vi "Initialize New.vi"(4 "Error In":errorcluster, 7 "Config Data_DB in":refnum<class "Config Data_DB.lvclass">) -> (0 "Error Out":errorcluster, 3 "Config Data_DB out":refnum<class "Config Data_DB.lvclass">)   [LabVIEW 2014, in "Config Data.lvlib" / "Config Data_DB.lvclass"]
uses:
  Config Data_DB.lvclass
  Config Data_DB.lvclass/Config Data_DB.ctl
  Config Data.lvclass
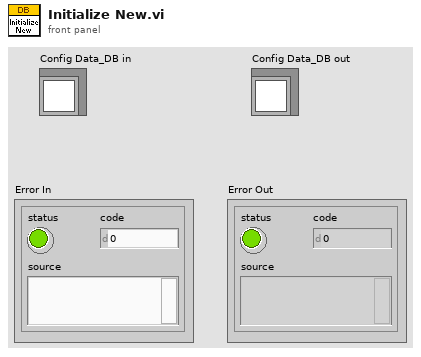
[diagram p1: front panel]
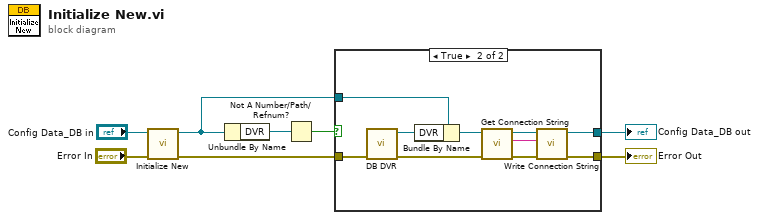
[diagram p0: block diagram]
diagram:
  n1 = call-parent "Initialize New.vi"("Error In"="Error In", "Config Data in"="Config Data_DB in") -> ("Error Out"=w3:errorcluster, "Config Data out"=w4:refnum<class "Config Data_DB.lvclass">)  [unwired: 4 in]
  n2 = Unbundle By Name(w4) -> ("DVR"=w6:refnum<data-value>)
  n3 = Not A Number/Path/Refnum?(number/path/refnum=w6) -> (NaN/Path/Refnum?=w5:bool)
  n4 = case shown="True" w5 {
    tunnel: w4 -> [w10 w20]
    tunnel: [w10 w12] -> w2
    tunnel: w3 -> [w9 w19]
    tunnel: [w9 w11] -> w1
    frame False {
    }
    frame True {
      n5 = call "DB DVR.vi"("Error In"=w19) -> ("Error Out"=w16:errorcluster, "DVR"=w18:refnum<data-value>)  [unwired: 5 in]
      n6 = Bundle By Name(cluster=w20, "DVR"=w18) -> (w17:refnum<class "Config Data_DB.lvclass">)
      n7 = call-dynamic "Get Connection String.vi"("Error In"=w16, "Config Data_DB in"=w17) -> ("Error Out"=w13:errorcluster, "Connection String"=w14:string, "Config Data_DB out"=w15:refnum<class "Config Data_DB.lvclass">)  [unwired: 3 in]
      n8 = call "Write Connection String.vi"("Error In"=w13, "Connection String"=w14, "DB In"=w15) -> ("Error Out"=w11:errorcluster, "DB Out"=w12:refnum<class "Config Data_DB.lvclass">)  [unwired: 3 in]
    }
  }
  "Error Out" <- w1
  "Config Data_DB out" <- w2
